vi "nearest_point.vi"(9 "point in":cluster{"y":dbl, "x":dbl}, 11 "Array in":T2(array[cluster])) -> (1 "centroid out":T1, 3 "distance output":dbl)   [LabVIEW 2016]
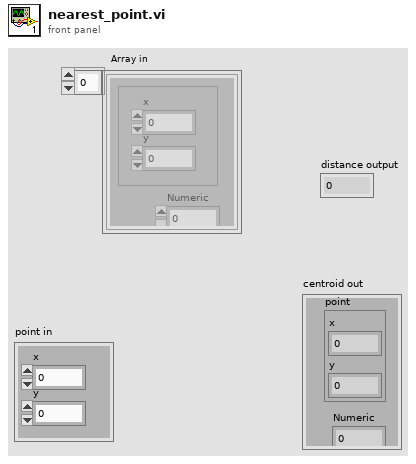
[diagram p1: front panel]
types:
  T1 = cluster{"point":cluster{"x":dbl, "y":dbl}, "Numeric":i32}
  T2 = cluster{"Cluster":cluster{"x":dbl, "y":dbl}, "Numeric":i32}[]
  T3 = cluster{"Cluster":cluster{"x":dbl, "y":dbl}, "Numeric":i32}
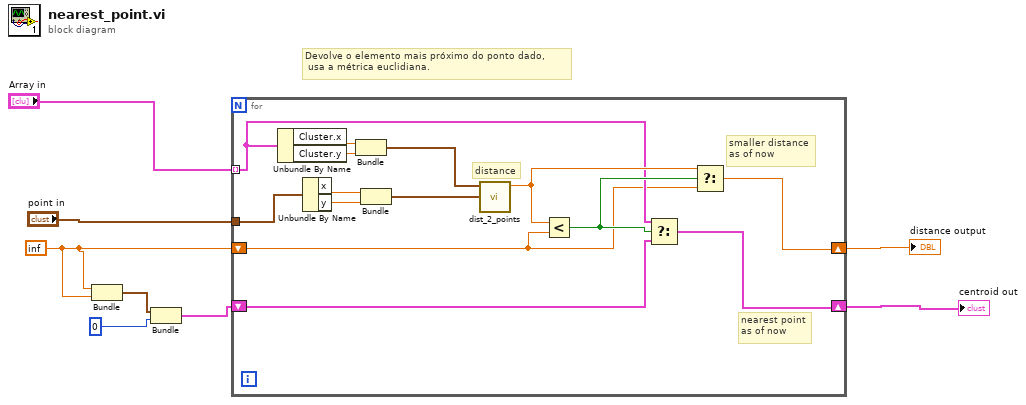
[diagram p0: block diagram]
diagram:
  w4 = inf
  # "Devolve o elemento mais próximo do ponto dado,\n usa a métrica euclidiana."
  n1 = Bundle(w4, w4) -> (w5:cluster{dbl, dbl})  [unwired: 1 in]
  n2 = Bundle(w5, 0) -> (w2:cluster{cluster{dbl, dbl}, i32})  [unwired: 1 in]
  n3 = for {
    tunnel: "Array in" -> [w10] mode=indexing
    tunnel: "point in" -> [w11]
    shift-right: [w18] -> w8
    shift-left: w4 -> [w9]
    shift-right: [w22] -> w6
    shift-left: w2 -> [w21]
    # "nearest point\nas of now"
    # "smaller distance\nas of now"
    # "distance"
    n4 = Unbundle By Name(w10) -> ("Cluster.x"=w16:dbl, "Cluster.y"=w17:dbl)
    n5 = Unbundle By Name(w11) -> ("x"=w13:dbl, "y"=w14:dbl)
    n6 = Bundle("x"=w16, "y"=w17) -> (w15:cluster{"x":dbl, "y":dbl})  [unwired: 1 in]
    n7 = Bundle("x"=w13, "y"=w14) -> (w12:cluster{"x":dbl, "y":dbl})  [unwired: 1 in]
    n8 = call "dist_2_points.vi"("point in 2"=w12, "point in 1"=w15) -> ("distance"=w19:dbl)  [unwired: 9 in]
    n9 = Less?(x=w19, y=w9) -> (x < y?=w20:bool)
    n10 = Select(t=w10, s=w20, f=w21) -> (s? t:f=w22:T3)
    n11 = Select(t=w19, s=w20, f=w9) -> (s? t:f=w18:dbl)
  }
  "distance output" <- w8
  "centroid out" <- w6
